vi "CreateSampleFilePaths.vi"(11 "Sample name":string) -> (1 "Sample directory path":path, 2 "Test sequence path":path, 4 "Log file path":path)   [LabVIEW 2013]
panel:
  out "error out":errorcluster
  in  "error in (no error)":errorcluster
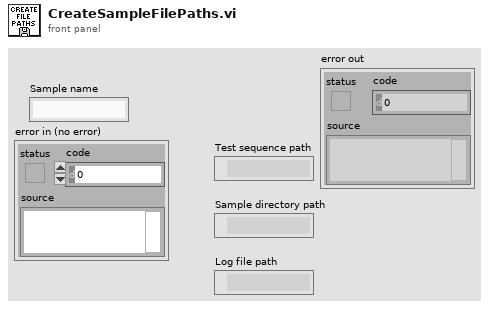
[diagram p1: front panel]
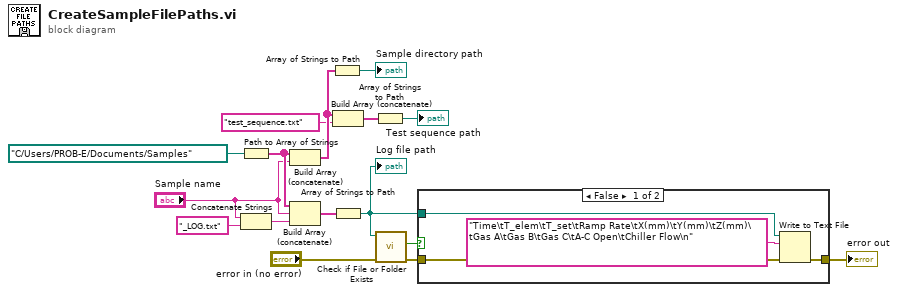
[diagram p0: block diagram]
diagram:
  n1 = Path to Array of Strings(0:path "C:/Users/PROB-E/Documents/Samples" ("Samples directory")) -> (2:w2:string[])  [unwired: 1 out]
  n2 = Concatenate Strings("Sample name", "_LOG.txt") -> (w11:string)
  n3 = Build Array (concatenate)(w2, "Sample name") -> (w15:string[])
  n4 = Build Array (concatenate)(w2, "Sample name", w11) -> (w9:string[])
  n5 = Array of Strings to Path(0:w15) -> (2:→"Sample directory path":path)  [unwired: 1 in]
  n6 = Build Array (concatenate)(w15, "test_sequence.txt") -> (w12:string[])
  n7 = Array of Strings to Path(0:w9) -> (2:w5:path)  [unwired: 1 in]
  "Log file path" <- w5
  n8 = Array of Strings to Path(0:w12) -> (2:→"Test sequence path":path)  [unwired: 1 in]
  n9 = call <vilib>:"Check if File or Folder Exists.vi"("error in (no error)"="error in (no error)", "path"=w5) -> ("error out"=w4:errorcluster, "file or folder exists?"=w6:bool)  [unwired: 7 in, 1 out]
  n10 = case shown="False" w6 {
    tunnel: w5 -> [w19 _]
    tunnel: w4 -> [w17 w21]
    tunnel: [w18 w21] -> w3
    frame False {
      n11 = Write to Text File(file (use dialog)=w19, text="Time\tT_elem\tT_set\tRamp Rate\tX(mm)\tY(mm)\tZ(mm)\tGas A\tGas B\tGas C\tA-C Open\tChiller Flow\n", error in=w17) -> (error out=w18:errorcluster)  [unwired: 1 in, 2 out]
    }
    frame True {
    }
  }
  "error out" <- w3
